vi "ArmInverseKinematics.vi"(5 "max steps":i32=100, 6 "joint constraints":cluster{dbl, dbl}[](array[cluster]), 7 "mask":dbl[](array[numeric]), 8 "error in (no error)":errorcluster, 9 "current joint positions":dbl[](array[numeric]), 10 "end effector transform":T1, 11 "serial arm in":refnum<class "NI_Robotics_Serial Robot Arm.lvclass">) -> (0 "error out":errorcluster, 1 "steps taken":i32, 2 "joint positions":dbl[](array[numeric]), 3 "serial arm out":refnum<class "NI_Robotics_Serial Robot Arm.lvclass">)   [LabVIEW 2020]
doc: "Computes the joint angles of a robotic arm given the location of the end effector relative to the arm base. Wire data to the <B>end effector transform</B> input to determine the polymorphic instance to use or manually select the instance.\n\n<B>.m file:</B> ikine"
uses:
  <vilib>/robotics/Kinematics/Robot/NI_Robotics_Serial Robot Arm.lvclass
  <vilib>/Analysis/Matrix/Datatypes/RealMatrix.ctl
  <vilib>/Analysis/_algsub.llb/Real Vector Norm.vi
  <vilib>/robotics/Kinematics/Transform2ToDiff.vi
  <vilib>/Analysis/7linalg.llb/Solve Linear Equations (single right hand).vi
  <vilib>/Analysis/baseanly.llb/Solve Linear Equations By Cholesky.vi
  <vilib>/Analysis/baseanly.llb/Real Matrix to Compact Array.vi
  <vilib>/Analysis/baseanly.llb/Real Compact Tri-Matrix Linear Eqs.vi
  <vilib>/Analysis/coordinate.llb/Cross Product.vi
  <vilib>/Analysis/7linalg.llb/Solve Linear Eqs (General).vi
  <vilib>/Analysis/7linalg.llb/Solve Linear Eqs (Gen, single right hand).vi
  <vilib>/robotics/Kinematics/NI_Kinematics.lvlib
  <vilib>/Analysis/NI_AALPro.lvlib
  <vilib>/robotics/Utilities/NI_Robotics Utilities.lvlib
  <vilib>/Analysis/Matrix/NI_Matrix.lvlib
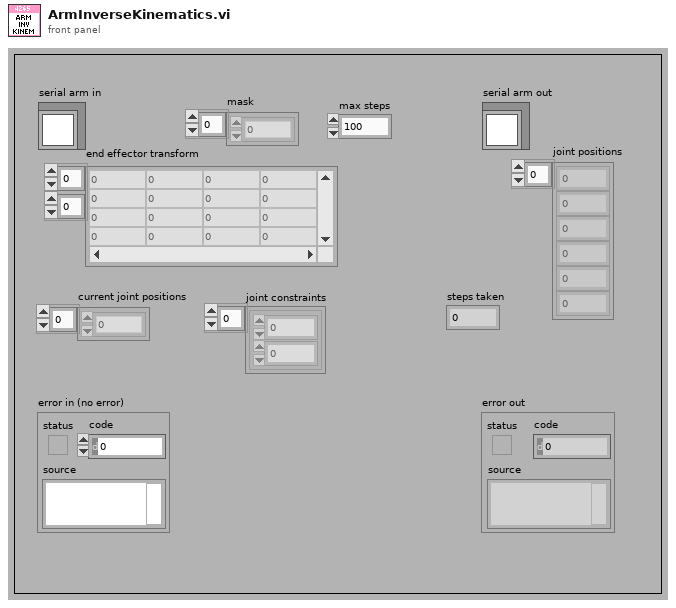
[diagram p1: front panel]
types:
  T1 = typedef "NI_Matrix.lvlib/RealMatrix.ctl" = dbl[][]
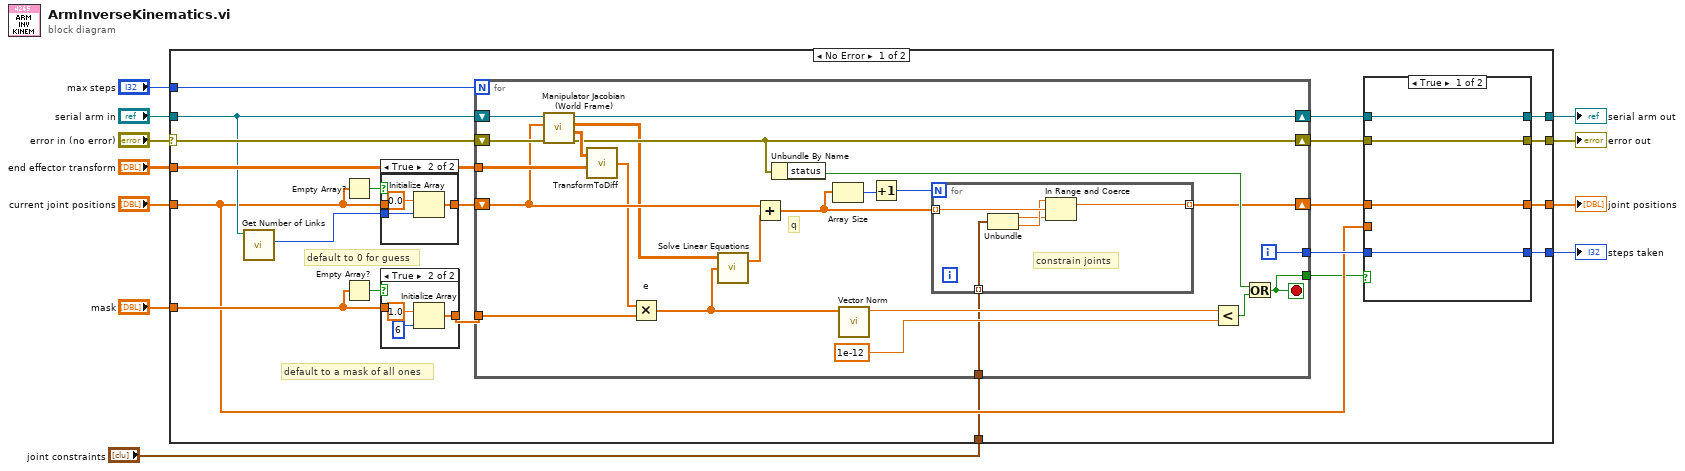
[diagram p0: block diagram]
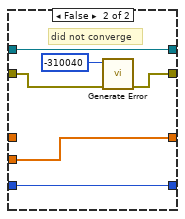
[diagram p2: hidden frame]
diagram:
  n1 = case shown="No Error" "error in (no error)" {
    selector: "error in (no error)" -> [w28 w81]
    tunnel: [w17 w81] -> w10
    tunnel: [w16 w80] -> w8
    tunnel: "serial arm in" -> [w24 w80]
    tunnel: "mask" -> [w31 _]
    tunnel: "current joint positions" -> [w14 w79]
    tunnel: "end effector transform" -> [w29 _]
    tunnel: [w19 w79] -> w4
    tunnel: [w21 _] -> w3
    tunnel: "max steps" -> [w23 _]
    tunnel: "joint constraints" -> [w12 _]
    frame No Error {
      # "default to a mask of all ones"
      # "default to 0 for guess"
      n2 = call <vilib>:"Get Number of Links.vi"("serial arm in"=w24) -> ("number of links"=w25:i32)  [unwired: 8 in, 2 out]
      n3 = Empty Array?(array=w14) -> (empty?=w27:bool)
      n4 = Empty Array?(array=w31) -> (empty?=w32:bool)
      n5 = case shown="True" w27 {
        tunnel: w14 -> [w43 _]
        tunnel: [w43 w44] -> w26
        tunnel: w25 -> [_ w45]
        frame False {
        }
        frame True {
          n6 = Initialize Array(0.0 ("element"), w45) -> (w44:dbl[])
        }
      }
      n7 = case shown="True" w32 {
        tunnel: w31 -> [w75 _]
        tunnel: [w75 w77] -> w30
        frame False {
        }
        frame True {
          n8 = Initialize Array(1.0 ("element"), 6 ("dimension size")) -> (w77:dbl[])
        }
      }
      n9 = for {
        N: w23 -> [_]
        tunnel: w30 -> [w69]
        shift-right: [w47] -> w20
        shift-left: w26 -> [w59]
        tunnel: w29 -> [w66]
        shift-right: [w62] -> w18
        shift-left: w28 -> [w64]
        shift-right: [w68] -> w15
        shift-left: w24 -> [w65]
        tunnel: [w57] -> w22
        tunnel: [w56] -> w13
        tunnel: w12 -> [w51]
        i -> [w57]
        stop <- w56 stop-if-true
        # "q"
        n10 = call <vilib>:"Manipulator Jacobian (World Frame).vi"("error in (no error)"=w64, "joint positions"=w59, "serial arm in"=w65) -> ("error out"=w62:errorcluster, "forward kinematics"=w63:T1, "jacobian"=w55:T1, "serial arm out"=w68:refnum<class "NI_Robotics_Serial Robot Arm.lvclass">)  [unwired: 5 out]
        n11 = call-poly <vilib>:"TransformToDiff.vi"("End Transform"=w66, "Start Transform"=w63) -> ("Differential"=w58:dbl[])
        n12 = Multiply "e"(x=w58, y=w69) -> (x*y=w53:dbl[])
        n13 = call-poly <vilib>:"Solve Linear Equations.vi"("Known Vector"=w53, "Input Matrix"=w55) -> ("Solution Vector"=w54:dbl[])  [unwired: 1 in, 1 out]
        n14 = Add ("Add.vi")(x=w59, y=w54) -> (x+y=w49:dbl[])
        n15 = Unbundle By Name(w62) -> ("status"=w60:bool)
        n16 = Array Size(array=w49) -> (size(s)=w50:i32)
        n17 = call-poly <vilib>:"Vector Norm.vi"("Input Vector"=w53) -> ("norm"=w52:dbl)  [unwired: 2 in, 8 out]
        n18 = Increment(x=w50) -> (x+1=w48:i32)
        n19 = for {
          N: w48 -> [_]
          tunnel: w49 -> [w74] mode=indexing
          tunnel: [w73] -> w47 mode=indexing
          tunnel: w51 -> [w72] mode=indexing
          # "constrain joints"
          n20 = Unbundle(w72) -> (w70:dbl, w71:dbl)
          n21 = In Range and Coerce(upper limit=w71, x=w74, lower limit=w70) -> (coerced(x)=w73:dbl)  [unwired: 1 out]
        }
        n22 = Less?(x=w52, y=1e-12 ("element")) -> (x < y?=w61:bool)
        n23 = Or(x=w60, y=w61) -> (x .or. y?=w56:bool)
      }
      n24 = case shown="True" w13 {
        tunnel: w22 -> [w33 w42]
        tunnel: [w33 w42] -> w21
        tunnel: w20 -> [w34 _]
        tunnel: [w34 w37] -> w19
        tunnel: w18 -> [w35 w39]
        tunnel: [w35 w38] -> w17
        tunnel: [w36 w41] -> w16
        tunnel: w15 -> [w36 w41]
        tunnel: w14 -> [_ w37]
        frame True {
        }
        frame False {
          # "did not converge"
          n25 = call <vilib>:"Generate Error.vi"("error in (no error)"=w39, "code"=-310040) -> ("error out"=w38:errorcluster)  [unwired: 9 in]
        }
      }
    }
    frame Error {
    }
  }
  "error out" <- w10
  "serial arm out" <- w8
  "joint positions" <- w4
  "steps taken" <- w3
